vi "TimeArrange.vi"(2 "Din":cluster{"时间(s)":dbl[], "数据":dbl[]}) -> (9 "Dout":cluster{"时间(s)":dbl[], "数据":dbl[]})   [LabVIEW 2015]
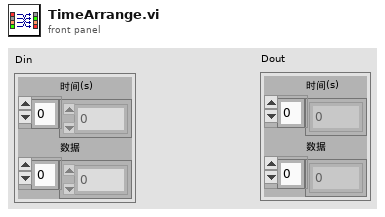
[diagram p1: front panel]
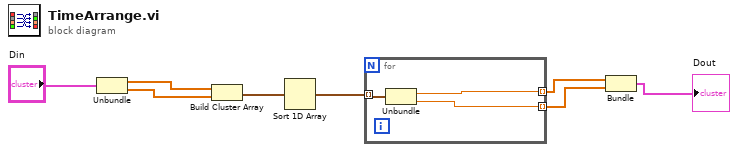
[diagram p0: block diagram]
diagram:
  n1 = Unbundle("Din") -> ("时间(s)"=w7:dbl[], "数据"=w6:dbl[])
  n2 = Build Cluster Array(w7, w6) -> (w5:cluster{dbl, dbl}[])
  n3 = Sort 1D Array(array=w5) -> (sorted array=w4:cluster{dbl, dbl}[])
  n4 = for {
    tunnel: w4 -> [w11] mode=indexing
    tunnel: [w10] -> w2 mode=indexing
    tunnel: [w9] -> w1 mode=indexing
    n5 = Unbundle(w11) -> (w10:dbl, w9:dbl)
  }
  n6 = Bundle(w2, w1) -> (→"Dout":cluster{dbl[], dbl[]})  [unwired: 1 in]
